vi "Mask Write Register.vi"(4 "OR Mask":u16, 6 "AND Mask":u16, 8 "error in":errorcluster, 10 "address":u16, 11 "device data model in":refnum<class "Standard Data Model.lvclass">) -> (0 "error out":errorcluster, 3 "device data model out":refnum<class "Standard Data Model.lvclass">)   [LabVIEW 2013, in "Modbus Library - Advance.lvlib" / "Standard Data Model.lvclass"]
doc: "Writes the masked value of a single register using an <b>AND mask</b> and an <b>OR mask</b> using the equation below:\nResult=(Current Value AND AndMask) OR (OrMask AND !AndMask)"
uses:
  Standard Data Model.lvclass
  Standard Data Model.lvclass/Standard Data Model.ctl
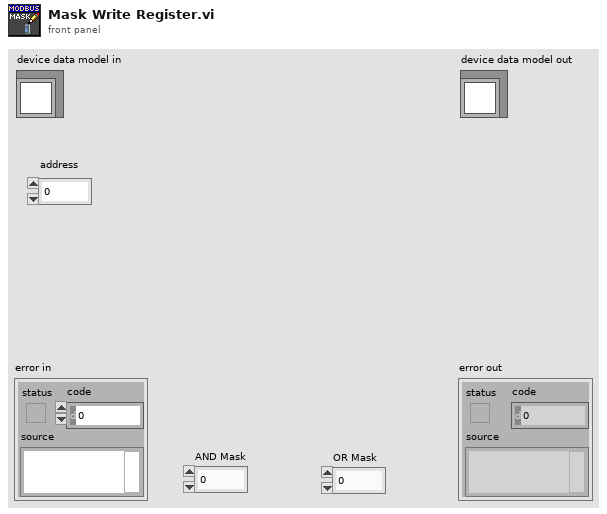
[diagram p1: front panel]
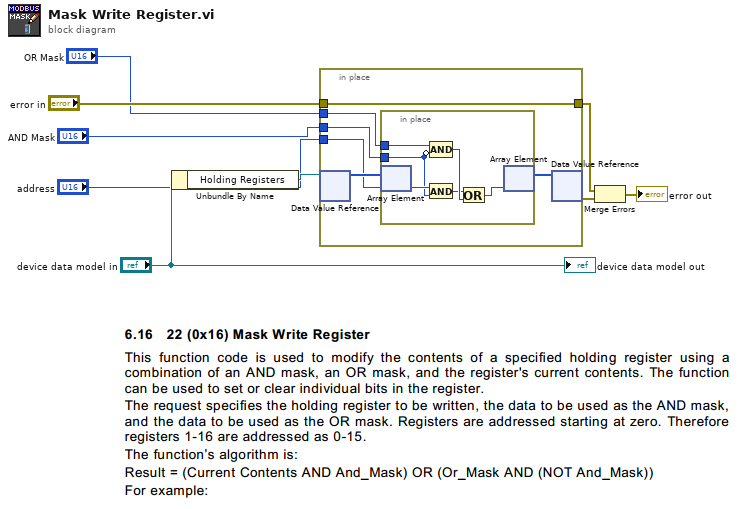
[diagram p0: block diagram]
diagram:
  n1 = Unbundle By Name("device data model in") -> ("Holding Registers"=w6:refnum<data-value>)
  n2 = in-place {
    in-place-border: "error in" -> [w15]
    in-place-border: [w15] -> w4
    in-place-border: "address" -> [w13]
    in-place-border: "AND Mask" -> [w11]
    in-place-border: "OR Mask" -> [w10]
    n3 = in-place-dvr #1(w6) -> (w14:u16[])  [unwired: 1 out]
    n4 = in-place {
      in-place-border: w11 -> [w17]
      in-place-border: w10 -> [w16]
      n5 = in-place-array #2(w14, w13) -> (w19:u16)
      n6 = And(x=w19, y=w17) -> (x .and. y?=w20:u16)
      n7 = Compound Arithmetic op=AND(w16, invert w17) -> (w21:u16)
      n8 = Or(x=w20, y=w21) -> (x .or. y?=w18:u16)
      n9 = in-place-array #2(w18) -> (w12:u16[])  [unwired: 1 out]
    }
    n10 = in-place-dvr #1(w12) -> (w5:errorcluster)  [unwired: 1 out]
  }
  n11 = Merge Errors(w4, w5) -> (→"error out":errorcluster)
  "device data model out" <- "device data model in"
